vi "UUT - Write Image Data.vi"(8 "error in (no error)":errorcluster, 9 "Simulation Data":T1={"PowerOn"=TRUE, "Battery"=TRUE, "Antenna"=TRUE, "Microphone"=TRUE, "Speakers"=TRUE, "Buttons"=TRUE, "LCD"=enum."Passing Image"}, 10 "Test Image Data":u32[][](array[numeric]), 11 "VISA resource name":refnum<visa-resource-name>) -> (0 "error out":errorcluster, 3 "VISA resource name out":refnum<visa-resource-name>)   [LabVIEW 2011]
uses:
  Simulation Data.ctl
  Video Hardware Simulation Commands.ctl
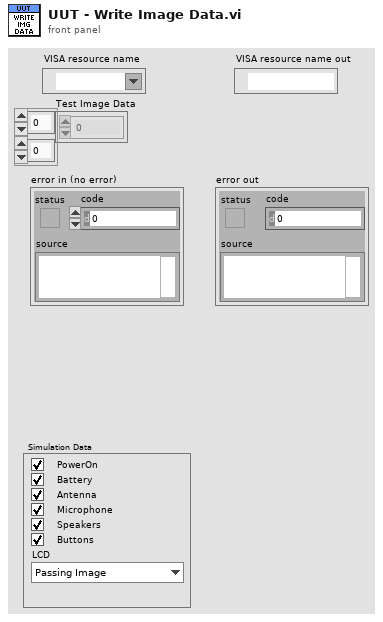
[diagram p1: front panel]
types:
  T1 = typedef "Simulation Data.ctl" = cluster{"PowerOn":bool, "Battery":bool, "Antenna":bool, "Microphone":bool, "Speakers":bool, "Buttons":bool, "LCD":enum16{"Passing Image", "Dead Pixels", "Incorrect Brightness"}}
  T2 = typedef "Video Hardware Simulation Commands.ctl" = enum16{"Simulate Generate Video Output", "Simulate Read HDMI Data"}
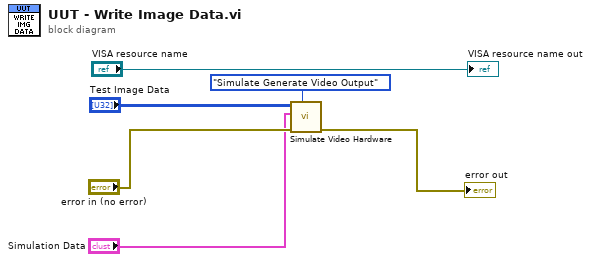
[diagram p0: block diagram]
diagram:
  n1 = call "Simulate Video Hardware.vi"("Command to Simulate"=Video_Hardware_Simulation_Commands."Simulate Generate Video Output", "error in (no error)"="error in (no error)", "Simulation Data"="Simulation Data", "Test Image Data"="Test Image Data") -> ("error out"=→"error out":errorcluster)  [unwired: 6 in, 1 out]
  "VISA resource name out" <- "VISA resource name"
